vi "RSZVB Get Sweep Segment Independent Time.vi"(8 "error in (no error)":errorcluster {"code" format="%.0x"}, 9 "Segment (1)":i32=1, 10 "Channel (1)":i32=1, 11 "VISA session":refnum<visa-resource-name>) -> (0 "error out":errorcluster {"code" format="%.0x"}, 2 "Time":bool, 3 "dup VISA session":refnum<visa-resource-name>)   [LabVIEW 2011]
doc: "This VI queries whether or not the Sweep Time can be set independently for each sweep segment.\n\nRemote-control command(s):\n[SENSe<Ch>:]SEGMent<Seg>:SWEep:TIME:CONTrol?"
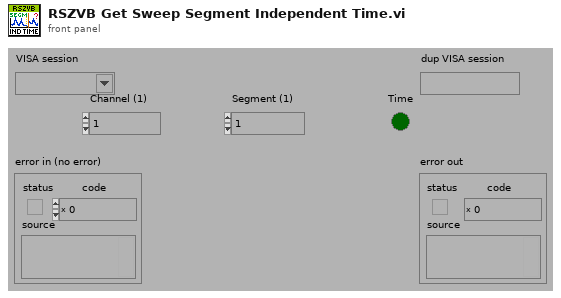
[diagram p1: front panel]
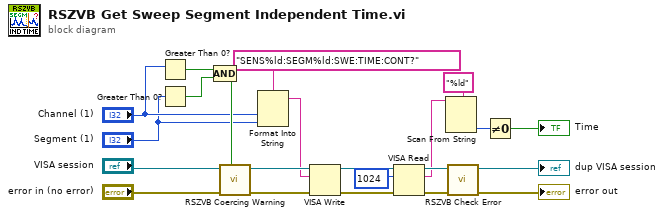
[diagram p0: block diagram]
diagram:
  n1 = Greater Than 0?(x="Channel (1)") -> (x > 0?=w17:bool)
  n2 = Greater Than 0?(x="Segment (1)") -> (x > 0?=w16:bool)
  n3 = Compound Arithmetic op=AND(w17, w16) -> (w19:bool)
  n4 = call "RSZVB Coercing Warning.vi"("In Range?"=w19, "error in (no error)"="error in (no error)", "VISA session"="VISA session") -> ("error out"=w20:errorcluster, "dup VISA session"=w21:refnum<visa-resource-name>)  [unwired: 7 in]
  n5 = Format Into String(format string="SENS%ld:SEGM%ld:SWE:TIME:CONT?", "Channel (1)", "Segment (1)") -> (resulting string=w18:string)  [unwired: 2 in, 1 out]
  n6 = VISA Write(VISA resource name=w21, write buffer=w18, error in (no error)=w20) -> (VISA resource name out=w9:refnum<visa-resource-name>, error out=w8:errorcluster)  [unwired: 1 out]
  n7 = VISA Read(VISA resource name=w9, byte count=u32 1024 ("byte count (0)"), error in (no error)=w8) -> (VISA resource name out=w14:refnum<visa-resource-name>, read buffer=w11:string, error out=w13:errorcluster)  [unwired: 1 out]
  n8 = Scan From String(format string="%ld", input string=w11) -> (output 1=w10:i32)  [unwired: 3 in, 3 out]
  n9 = call "RSZVB Check Error.vi"("error in (no error)"=w13, "VISA session"=w14) -> ("error out"=→"error out":errorcluster, "dup VISA session"=→"dup VISA session":refnum<visa-resource-name>)  [unwired: 8 in]
  n10 = Not Equal To 0?(x=w10) -> (x != 0?=→"Time":bool)
